vi "Sensirion SHT25 - VISA read user register.vi"(8 "Error In":errorcluster, 11 "VISA in":refnum<visa-resource-name>) -> (0 "Error Out":errorcluster, 1 "user register":u8 format="%08b", 3 "VISA out":refnum<visa-resource-name>)   [LabVIEW 2012]
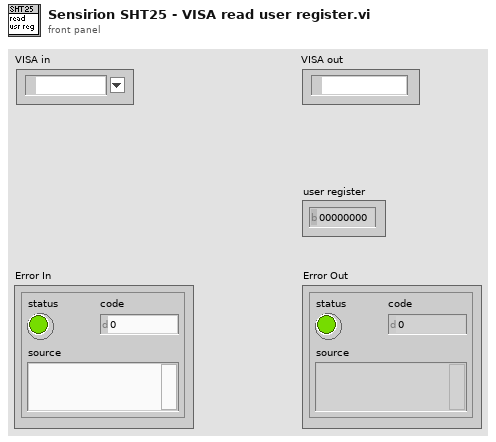
[diagram p1: front panel]
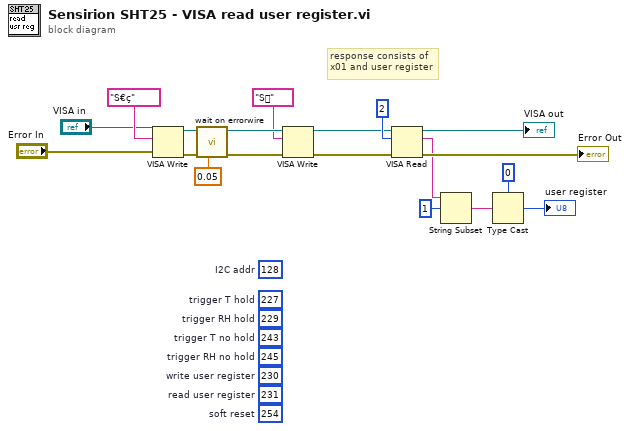
[diagram p0: block diagram]
diagram:
  (unwired) u8 254  # soft reset
  (unwired) u8 231  # read user register
  (unwired) u8 230  # write user register
  (unwired) u8 245  # trigger RH no hold
  (unwired) u8 243  # trigger T no hold
  (unwired) u8 229  # trigger RH hold
  (unwired) u8 128  # I2C addr
  (unwired) u8 227  # trigger T hold
  # "response consists of\nx01 and user register"
  n1 = VISA Write(VISA resource name="VISA in", write buffer="S€ç", error in (no error)="Error In") -> (VISA resource name out=w10:refnum<visa-resource-name>, error out=w14:errorcluster)  [unwired: 1 out]
  n2 = call "wait on errorwire.vi"("Delay Time (s)"=0.05, "error in (no error)"=w14) -> ("error out"=w9:errorcluster)  [unwired: 9 in]
  n3 = VISA Write(VISA resource name=w10, write buffer="S", error in (no error)=w9) -> (VISA resource name out=w7:refnum<visa-resource-name>, error out=w8:errorcluster)  [unwired: 1 out]
  n4 = VISA Read(VISA resource name=w7, byte count=u32 2, error in (no error)=w8) -> (VISA resource name out=→"VISA out":refnum<visa-resource-name>, read buffer=w5:string, error out=→"Error Out":errorcluster)  [unwired: 1 out]
  n5 = String Subset(string=w5, offset (0)=1) -> (substring=w3:string)  [unwired: 1 in]
  n6 = Type Cast(type=u8 0 ("element"), x=w3) -> (*(type *) &x=→"user register":u8)
